vi "FA_Apply.vi"(8 "Error In":errorcluster, 11 "Special Type":T1) -> (0 "Error Out":errorcluster)   [LabVIEW 2014, in "FA_ApplySysConfig.lvlib"]
uses:
  FA_ApplySysConfig.lvlib
  FA_LocalStore API/source/VI Source/FA_LocalStore.lvlib
  FA_LocalStore API/source/VI Source/FA_LSCollections.ctl
  Shared Code/AMC/VI Source/CentralProcessMessaging/Flock_Shared_CentralProcessMessaging.lvlib
  FA_LocalStore API/source/VI Source/FA_LSSpecialTypes.ctl
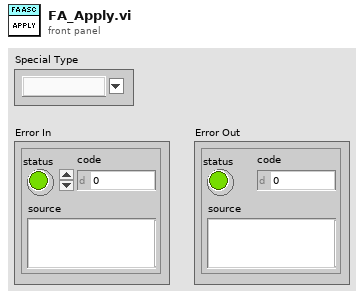
[diagram p1: front panel]
types:
  T1 = typedef "FA_LocalStore.lvlib/FA_LSSpecialTypes.ctl" = string
  T2 = typedef "FA_LocalStore.lvlib/FA_LSCollections.ctl" = enum16{"Config", "ConfigItem", "FA_eTag", "FA_PlugIn"}
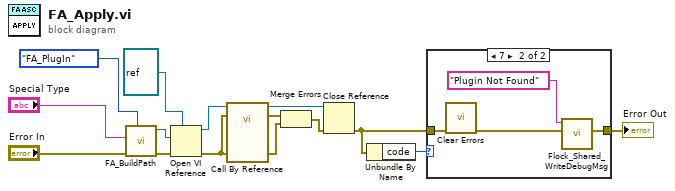
[diagram p0: block diagram]
diagram:
  n1 = call "FA_BuildPath.vi"("LSCollections"=FA_LSCollections."FA_PlugIn", "error in (no error)"="Error In", "Special Type"="Special Type") -> ("error out"=w12:errorcluster, "file path"=w14:path)  [unwired: 6 in, 1 out]
  n2 = Open VI Reference(type specifier VI Refnum (for type only)=refnum<vi> refnum, vi path=w14, error in (no error)=w12) -> (vi reference=w5:refnum<vi>, error out=w10:errorcluster)  [unwired: 3 in]
  n3 = call-by-ref "?"(reference=w5, error in=w10, "Error In"=w10) -> (reference out=w7:refnum<vi>, error out=w9:errorcluster, "Error Out"=w8:errorcluster)  [unwired: 10 in]
  n4 = Merge Errors(w9, w8) -> (w6:errorcluster)
  n5 = Close Reference(reference=w7, error in (no error)=w6) -> (error out=w3:errorcluster)
  n6 = Unbundle By Name(w3) -> ("code"=w2:i32)
  n7 = case shown="7" w2 {
    tunnel: w3 -> [w16 w20]
    tunnel: [w16 w18] -> w1
    frame 0, Default {
    }
    frame 7 {
      n8 = call <vilib>:"Clear Errors.vi"("error in (no error)"=w20) -> ("error out"=w19:errorcluster)  [unwired: 5 in, 1 out]
      n9 = call "Flock_Shared_WriteDebugMsg.vi"("error in (no error)"=w19, "Current Message Case"="Plugin Not Found") -> ("error out"=w18:errorcluster)  [unwired: 9 in]
    }
  }
  "Error Out" <- w1
